vi "WriteClassAttributeOld.vi"(5 "error in (no error)":errorcluster) -> (19 "error out":errorcluster)   [LabVIEW 2020, in "G#MethodTemplates.lvclass"]
uses:
  G#MethodTemplates.lvclass
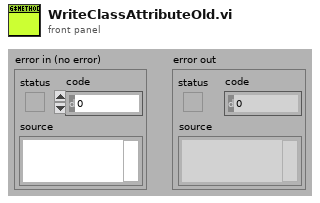
[diagram p1: front panel]
types:
  T1 = typedef "G#MethodTemplates.lvclass/ClassAttributes.ctl" = cluster{"Dummy":bool}
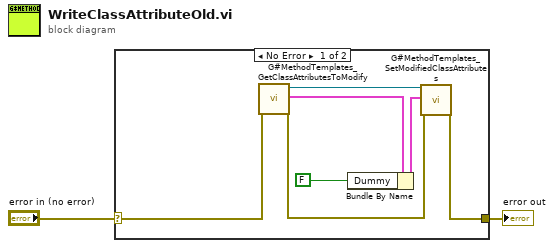
[diagram p0: block diagram]
diagram:
  n1 = case shown="No Error" "error in (no error)" {
    selector: "error in (no error)" -> [w4 w10]
    tunnel: [w7 w10] -> w1
    frame No Error {
      n2 = call "G#MethodTemplates_GetClassAttributesToModify.vi"("error in (no error)"=w4) -> ("reference out"=w8:refnum<class "G#BaseTemplateG3.lvclass">, "class attributes"=w3:T1, "error out"=w6:errorcluster)  [unwired: 13 in, 3 out]
      n3 = Bundle By Name(cluster=w3, "Dummy"=FALSE ("classAttribute1")) -> (w9:T1)
      n4 = call "G#MethodTemplates_SetModifiedClassAttributes.vi"("reference in"=w8, "attributes"=w9, "error in (no error)"=w6) -> ("error out"=w7:errorcluster)  [unwired: 15 in, 1 out]
    }
    frame Error {
    }
  }
  "error out" <- w1
